vi "DebugStateTimes2010.vi"(5 "ShowGUI":bool, 7 "reset":bool, 8 "error in":errorcluster, 11 "iteration":i32) -> (0 "error out":errorcluster, 3 "Current data":i32[][](array[numeric]))   [LabVIEW 2010]
doc: "This VI tracks the duration of execution based on an iteration index, use it to spot where an unknown wait is stalling your software.\nFor best results make sure this VI is called first in every state by using the Error in/out connections.\n\nUse <B>reset</B> to reinitialize the statistics\nUse <B>Show GUI</B> to open the dialog of the VI and present a sortable table."
uses:
  data/CM_SortableTable.xctl
  TableXControl/SortableTable.xctl
panel:
  out "Statistics (ms)":dbl[][](xcontrol)
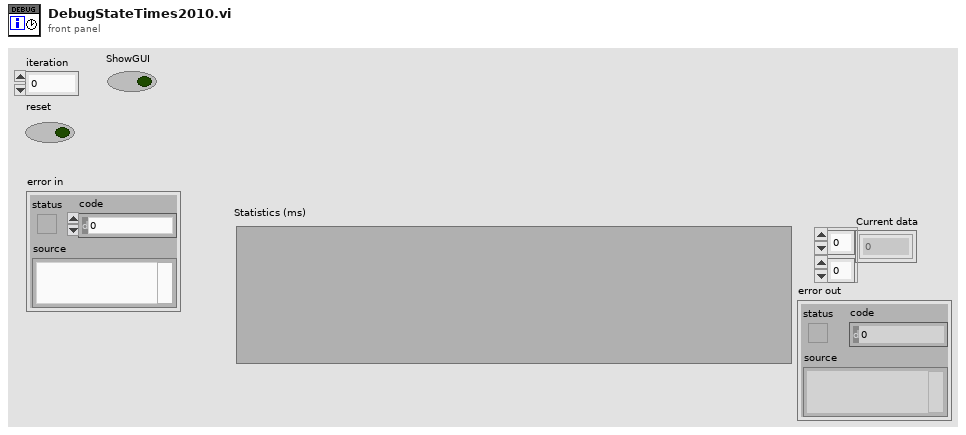
[diagram p1: front panel]
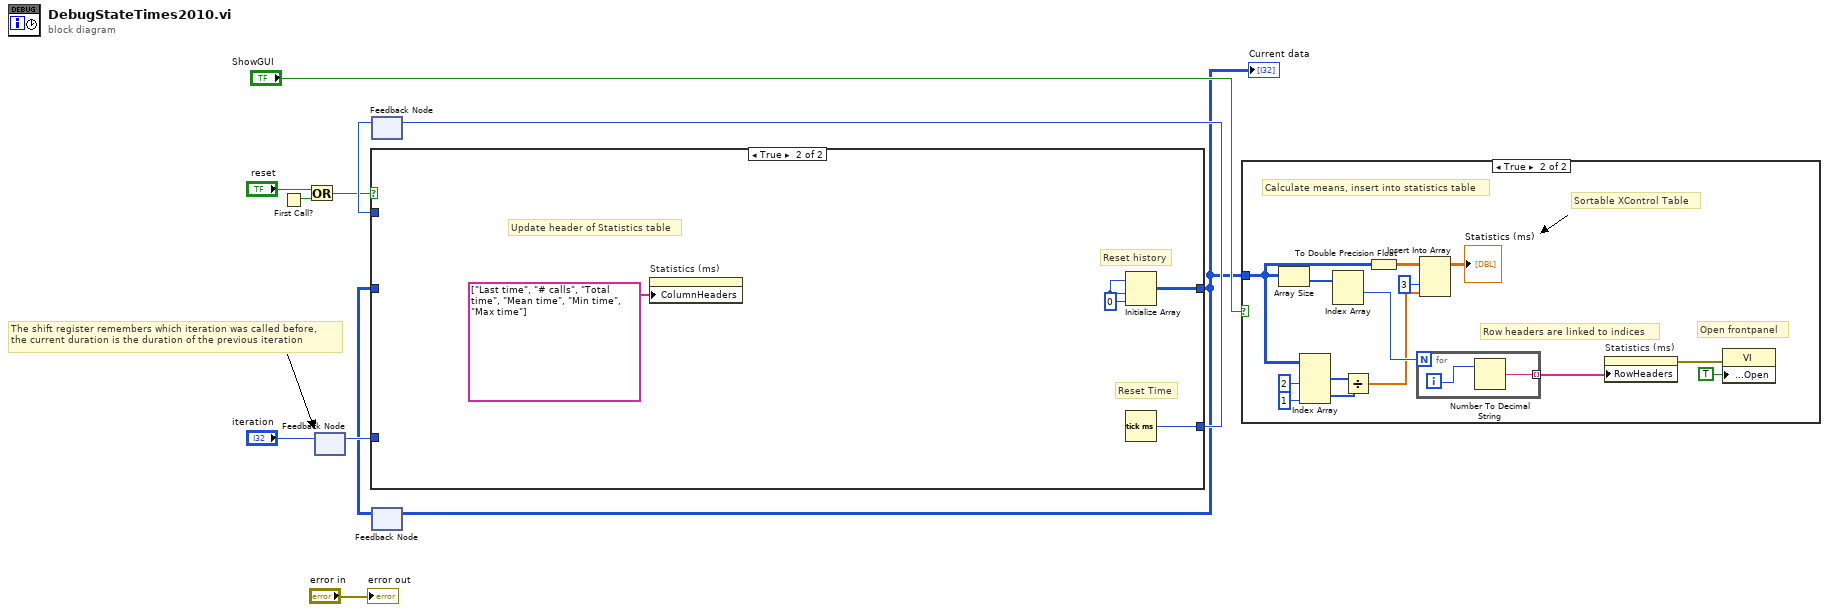
[diagram p0: block diagram]
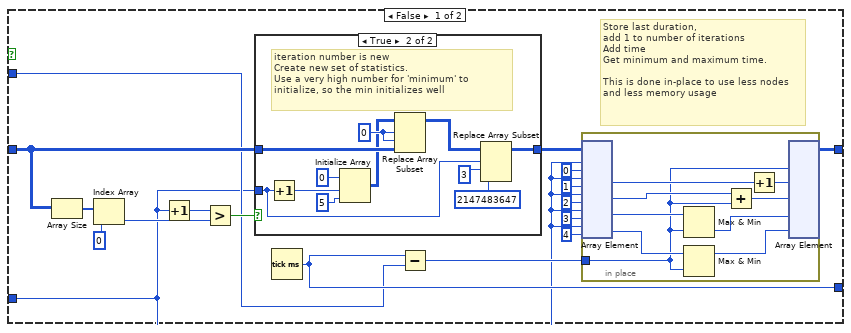
[diagram p3: hidden frame]
diagram:
  # "The shift register remembers which iteration was called before,\nthe current duration is the duration of the previous iteration"
  n1 = First Call?() -> (First Call?: T/F=w4:bool)
  n2 = Or(x="reset", y=w4) -> (x .or. y?=w2:bool)
  n3 = feedback #1() -> (w9:i32)  [unwired: 1 in]
  n4 = feedback-in #1("iteration") -> ()
  n5 = feedback #2() -> (w10:u32)  [unwired: 1 in]
  n6 = feedback #3() -> (w8:i32[][])  [unwired: 1 in]
  n7 = case shown="False" w2 {
    tunnel: [w19 w52] -> w5
    tunnel: w10 -> [w21 _]
    tunnel: [w27 w53] -> w11
    tunnel: w9 -> [w17 _]
    tunnel: w8 -> [w28 _]
    frame False {
      # "Store last duration,\nadd 1 to number of iterations\nAdd time\nGet minimum and maximum time.\n\nThis is done in-place to use less nodes\nand less memory usage"
      n8 = Array Size(array=w28) -> (size(s)=w25:i32[])
      n9 = Index Array(array=w25, index=0) -> (element=w24:i32)
      n10 = Increment(x=w17) -> (x+1=w22:i32)
      n11 = Greater?(x=w22, y=w24) -> (0:w26:bool)
      n12 = case shown="True" w26 {
        tunnel: w17 -> [_ w39]
        tunnel: w28 -> [w38 w47]
        tunnel: [w38 w41] -> w20
        frame False {
          # "Iteration number is allready known,\nreturn the current statistics"
        }
        frame True {
          w46 = 0 ("disabled index (col)")
          # "iteration number is new\nCreate new set of statistics.\nUse a very high number for 'minimum' to initialize, so the min initializes well"
          n13 = Increment(x=w39) -> (x+1=w44:i32)
          n14 = Initialize Array(0, w44, 5 ("dimension size")) -> (w45:i32[][])
          n15 = Replace Array Subset(array=w45, new element=w47, index (row)=w46, index (col)=w46) -> (w42:i32[][])
          n16 = Replace Array Subset(array=w42, new element=2147483647 ("new element/subarray"), index (row)=w39, index (col)=3 ("index")) -> (w41:i32[][])
        }
      }
      n17 = Tick Count (ms)() -> (millisecond timer value=w27:u32)
      n18 = Subtract(x=w27, y=w21) -> (x-y=w18:u32)
      n19 = in-place {
        in-place-border: w18 -> [w30]
        n20 = in-place-array #4(w20, w17, 0, w17, 1, w17, 2, w17, 3, w17, 4) -> (w37:i32, w35:i32, w33:i32, w31:i32)  [unwired: 1 out]
        n21 = Max & Min(x=w33, y=w30) -> (min(x,y)=w32:u32)  [unwired: 1 out]
        n22 = Max & Min(x=w31, y=w30) -> (max(x,y)=w29:u32)  [unwired: 1 out]
        n23 = Add(x=w35, y=w30) -> (x+y=w34:u32)
        n24 = Increment(x=w37) -> (x+1=w36:i32)
        n25 = in-place-array #4(w30, w36, w34, w32, w29) -> (w19:i32[][])  [unwired: 10 out]
      }
    }
    frame True {
      w51 = 0 ("dimension size")
      # "Update header of Statistics table"
      # "Reset history"
      # "Reset Time"
      n26 = property on="Statistics (ms)" class="SortableTable (strict)"("ColumnHeaders"=string[] ["Last time", "# calls", "Total time", "Mean time", "Min time", "Max time"]) -> ()  [unwired: 2 in, 2 out]
      n27 = Initialize Array(w51, w51, w51) -> (w52:i32[][])
      n28 = Tick Count (ms)() -> (millisecond timer value=w53:u32)
    }
  }
  "Current data" <- w5
  n29 = feedback-in #2(w11) -> ()
  n30 = feedback-in #3(w5) -> ()
  n31 = case shown="True" "ShowGUI" {
    tunnel: w5 -> [_ w55]
    frame False {
    }
    frame True {
      # "Open frontpanel"
      # "Sortable XControl Table"
      # "Calculate means, insert into statistics table"
      # "Row headers are linked to indices"
      n32 = Array Size(array=w55) -> (size(s)=w67:i32[])
      n33 = Index Array(array=w55, index (col) #1=2 ("disabled index (col)"), index (col) #2=1 ("index (col)")) -> (element #1=w64:i32[], element #2=w63:i32[])  [unwired: 2 in]
      n34 = Index Array(array=w67) -> (element #1=w62:i32)  [unwired: 2 in, 1 out]
      n35 = Divide(x=w64, y=w63) -> (x/y=w59:dbl[])
      n36 = To Double Precision Float(number=w55) -> (double precision float=w58:dbl[][])
      n37 = for {
        N: w62 -> [_]
        tunnel: [w69] -> w61 mode=indexing
        i -> [w68]
        n38 = Number To Decimal String(number=w68) -> (decimal integer string=w69:string)  [unwired: 1 in]
      }
      n39 = Insert Into Array(array=w58, index (col)=3 ("disabled index (col)"), new element=w59) -> (→"Statistics (ms)":dbl[][])  [unwired: 1 in]
      n40 = property on="Statistics (ms)" class="SortableTable (strict)"("RowHeaders"=w61) -> (error out=w54:errorcluster)  [unwired: 2 in, 1 out]
      n41 = property class="VI"(error in=w54, "Front Panel.Open"=TRUE ("Front Panel Window:Open")) -> ()  [unwired: 1 in, 2 out]
    }
  }
  "error out" <- "error in"
